vi "BM_Runze_Syringe_Pump_Controller.vi"(7 "Initialize Plunger?":bool, 8 "error in (no error)":errorcluster, 10 "COM Port (Runze)":refnum<visa-resource-name>="COM12" caption="COM Port", 11 "Enter Command":string="V150O1P19200O9V450D19200V150P23040O15V450D23040") -> (0 "error out":errorcluster={"status"=FALSE, "code"=1073676294, "source"="VISA Read in BM_Runze_Syringe_Pump_Controller.vi"}, 2 "Status":bool=TRUE, 3 "Response":string="`")   [LabVIEW 2021]
uses:
  <vilib>/Instr/_visa.llb/VISA Configure Serial Port (Instr).vi
panel:
  out "read buffer":string
  in  "Conversion factor\n(48000 steps/25 mL)":dbl=1920.0
  in  "Calculate Steps Needed":bool
  out "Steps Needed":dbl=23040.0
  in  "Volume desired (mL)":dbl=12.0
  out "Command":string="/1N1V150O1P19200O9V450D19200V150P23040O15V450D23040R\r"
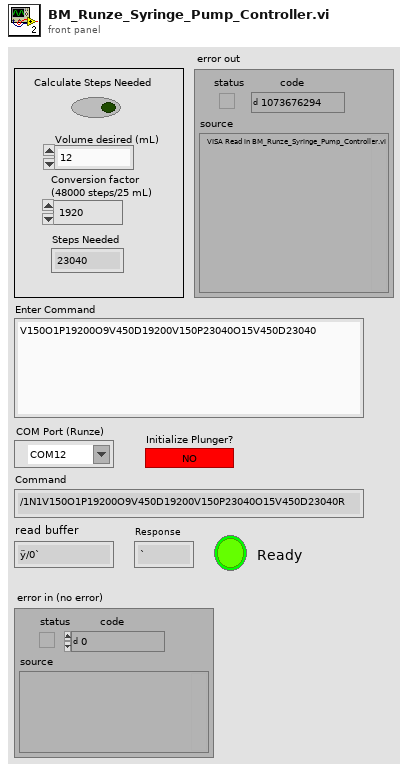
[diagram p1: front panel]
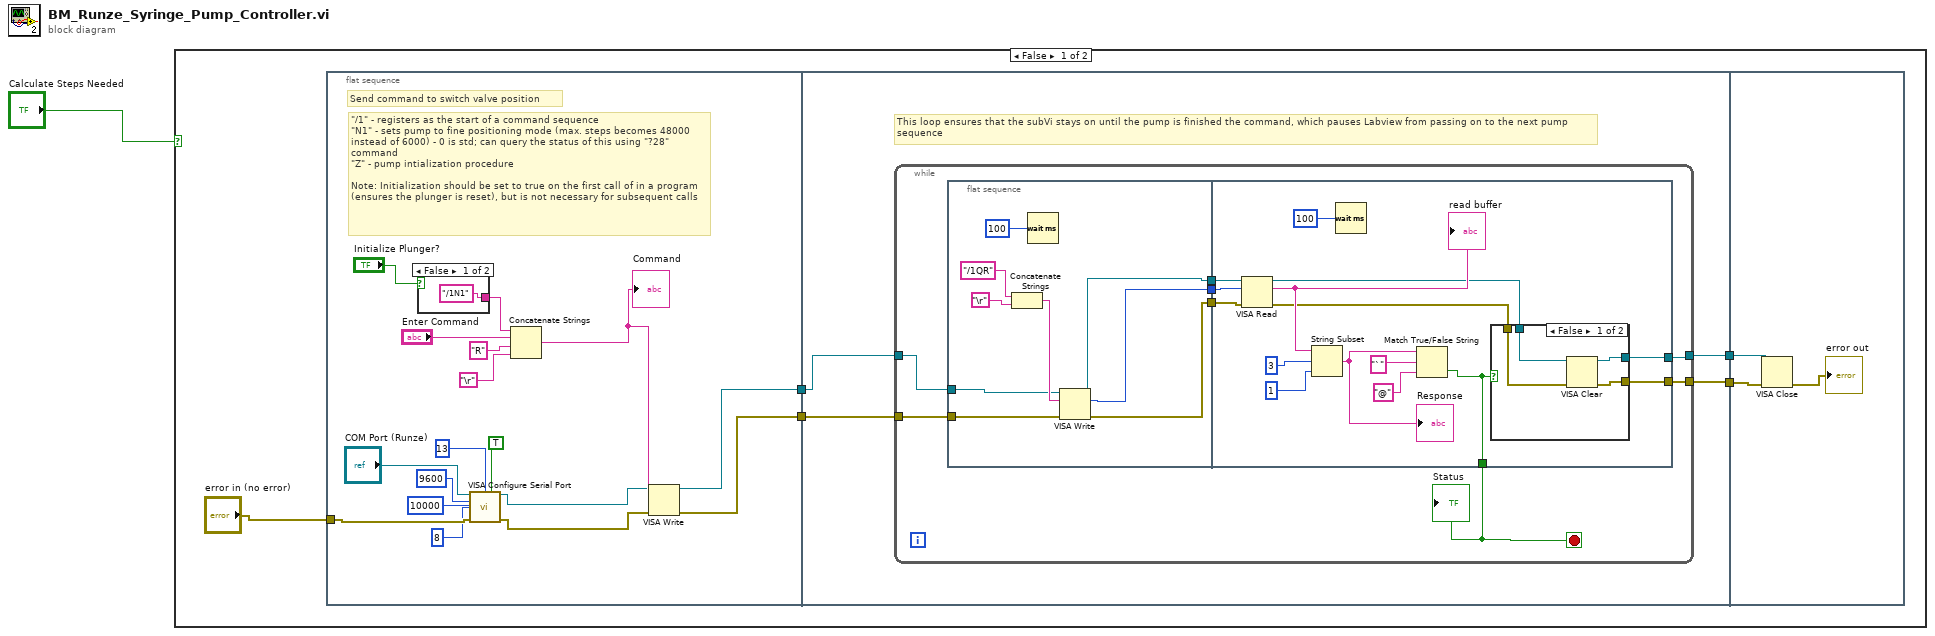
[diagram p0: block diagram]
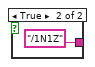
[diagram p2: hidden frame]
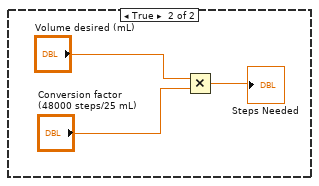
[diagram p4: hidden frame]
diagram:
  n1 = case shown="False" "Calculate Steps Needed" {
    frame False {
      n2 = flat-sequence {
        tunnel: [w22] -> w5
        tunnel: "error in (no error)" -> [w17]
        tunnel: [w16] -> w3
        tunnel: [w27] -> w6
        tunnel: w5 -> [w29]
        tunnel: w3 -> [w28]
        tunnel: [w26] -> w2
        tunnel: w6 -> [w69]
        tunnel: w2 -> [w68]
        frame #0 {
          # "\"/1\" - registers as the start of a command sequence\n\"N1\" - sets pump to fine positioning mode (max. steps becomes 48000 instead of 6000) - 0 is std; can query the status of this using \"?28\" command\n\"Z\" - pump intialization procedure\n\nNote: Initialization should be set to true on the first call of in a program (ensures the plunger is reset), but is not necessary for subsequent calls"
          # "Send command to switch valve position"
          n3 = case shown="False" "Initialize Plunger?" {
            tunnel: ["/1N1" ("string") "/1N1Z" ("string")] -> w18
            frame False {
            }
            frame True {
            }
          }
          n4 = call-poly "VISA Configure Serial Port"("VISA resource name"="COM Port (Runze)", "timeout (10sec)"=u32 10000, "termination char\n(0xA = '\\n' = LF)"=u8 13 ("termination char\n(0xA = '\\n' = LF)"), "Enable Termination\nChar (T)"=TRUE ("Enable Termination\nChar (T)"), "baud rate (9600)"=u32 9600, "data bits (8)"=u16 8, "error in (no error)"=w17) -> ("VISA resource name out"=w9:refnum<visa-resource-name>, "error out"=w8:errorcluster)  [unwired: 2 in, 5 out]
          n5 = Concatenate Strings(w18, "Enter Command", "R" ("string"), "\r") -> (w20:string)
          "Command" <- w20
          n6 = VISA Write(VISA resource name=w9, write buffer=w20, error in (no error)=w8) -> (VISA resource name out=w22:refnum<visa-resource-name>, error out=w16:errorcluster)  [unwired: 1 out]
        }
        frame #1 {
          # "This loop ensures that the subVi stays on until the pump is finished the command, which pauses Labview from passing on to the next pump sequence"
          n7 = while {
            tunnel: [w35] -> w26
            tunnel: w28 -> [w34]
            tunnel: w29 -> [w33]
            tunnel: [w36] -> w27
            stop <- w32 stop-if-true
            n8 = flat-sequence {
              tunnel: [w38] -> w37
              tunnel: w34 -> [w41]
              tunnel: w33 -> [w42]
              tunnel: [w40] -> w31
              tunnel: [w39] -> w30
              tunnel: w37 -> [w54]
              tunnel: [w52] -> w35
              tunnel: [w51] -> w36
              tunnel: [w50] -> w32
              tunnel: w31 -> [w55]
              tunnel: w30 -> [w56]
              frame #0 {
                n9 = Concatenate Strings("/1QR" ("write buffer"), "\r") -> (w44:string)
                n10 = Wait (ms)(milliseconds to wait=u32 100) -> ()  [unwired: 1 out]
                n11 = VISA Write(VISA resource name=w42, write buffer=w44, error in (no error)=w41) -> (VISA resource name out=w39:refnum<visa-resource-name>, return count=w38:u32, error out=w40:errorcluster)
              }
              frame #1 {
                n12 = VISA Read(VISA resource name=w56, byte count=w54, error in (no error)=w55) -> (VISA resource name out=w47:refnum<visa-resource-name>, read buffer=w57:string, error out=w48:errorcluster)  [unwired: 1 out]
                "read buffer" <- w57
                n13 = String Subset(string=w57, offset (0)=3, length (rest)=1) -> (substring=w53:string)
                "Response" <- w53
                n14 = Wait (ms)(milliseconds to wait=u32 100) -> ()  [unwired: 1 out]
                n15 = Match True/False String(2:"@", 3:"`", 4:w53) -> (0:w50:bool)  [unwired: 1 out]
                n16 = case shown="False" w50 {
                  tunnel: [w65 w66] -> w51
                  tunnel: [w64 w67] -> w52
                  tunnel: w48 -> [w63 w67]
                  tunnel: w47 -> [w62 w66]
                  frame False {
                    n17 = VISA Clear(VISA resource name=w62, error in (no error)=w63) -> (VISA resource name out=w65:refnum<visa-resource-name>, error out=w64:errorcluster)
                  }
                  frame True {
                  }
                }
              }
            }
            "Status" <- w32
          }
        }
        frame #2 {
          n18 = VISA Close(VISA resource name=w69, error in (no error)=w68) -> (error out=→"error out":errorcluster)
        }
      }
    }
    frame True {
      n19 = Multiply(x="Volume desired (mL)", y="Conversion factor\n(48000 steps/25 mL)") -> (x*y=→"Steps Needed":dbl)
    }
  }
